vi "G# - InterfaceDemo3.vi"() -> ()   [LabVIEW 2017]
doc: "G# Interface Implementation\nThis examples demonstrates how to use the G#Interface. The interface concept is an alternative design principle to multiple inheritance (just as in C# and Java). Classes that are not related can implement the same interface and the reference of the interface could be treated just as they are from the same class.\n\nBy using the G# Debugger found in Tools->G# Debugger a text log can be followed showing how the objects were created and destroyed."
uses:
  IMyInterface2_interface/IMyInterface2.lvclass
  C:/Program Files (x86)/National Instruments/LabVIEW 2017/vi.lib/addons/_AddQ/G#Object/G#Object.lvclass
  MyClass3_class/MyClass3.lvclass
  <vilib>/addons/_AddQ/G#Object/G#Object.lvclass
  MyClass4_class/MyClass4.lvclass
panel:
  out "# of objects killed":i32
  out "OK":bool
  in  "error in (no error)":errorcluster
  out "MyClass4 is instance of IMyInterface":bool
  out "MyClass3 is instance of IMyInterface":bool
  out "error out":errorcluster
  out "Class Name":string[](array[string])
  # "G# Interface Implementation without wrapper classes using dependecy injection\nThis examples demonstrates how to use the G#Interface without using wrapper classes. It also uses dependency injection to inject the implementing class to the interface.\nThe interface concept is an alternative design principle to multiple inheritance (just as in C# and Java).\nClasses that are not related can implement the same interface and the reference of the interface could be treated just as they are from the same class.\n\nBy using the G# Debugger found in Tools->G# Debugger a text log can be followed showing how the objects were created and destroyed."
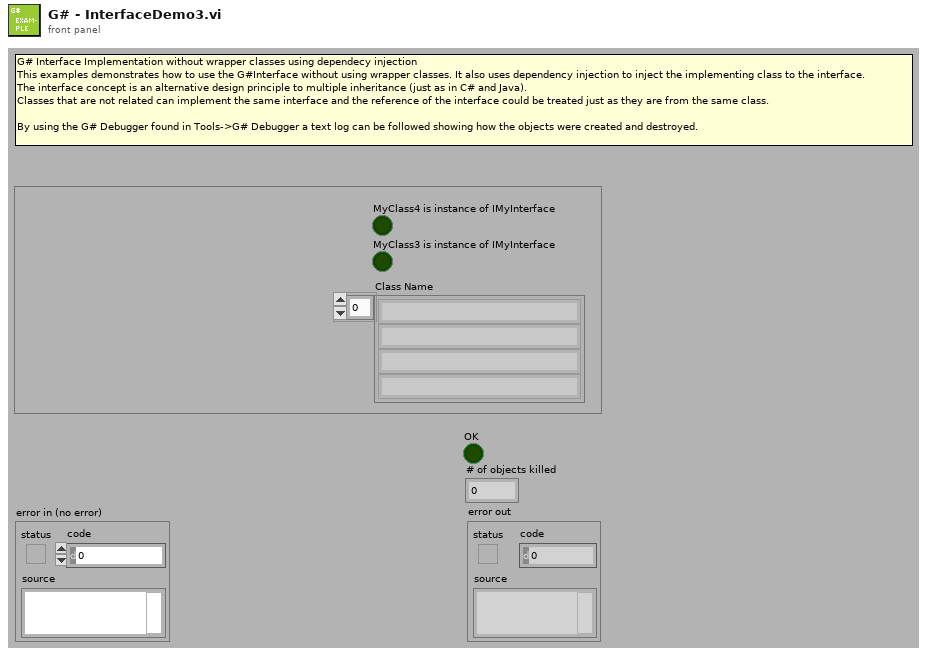
[diagram p1: front panel]
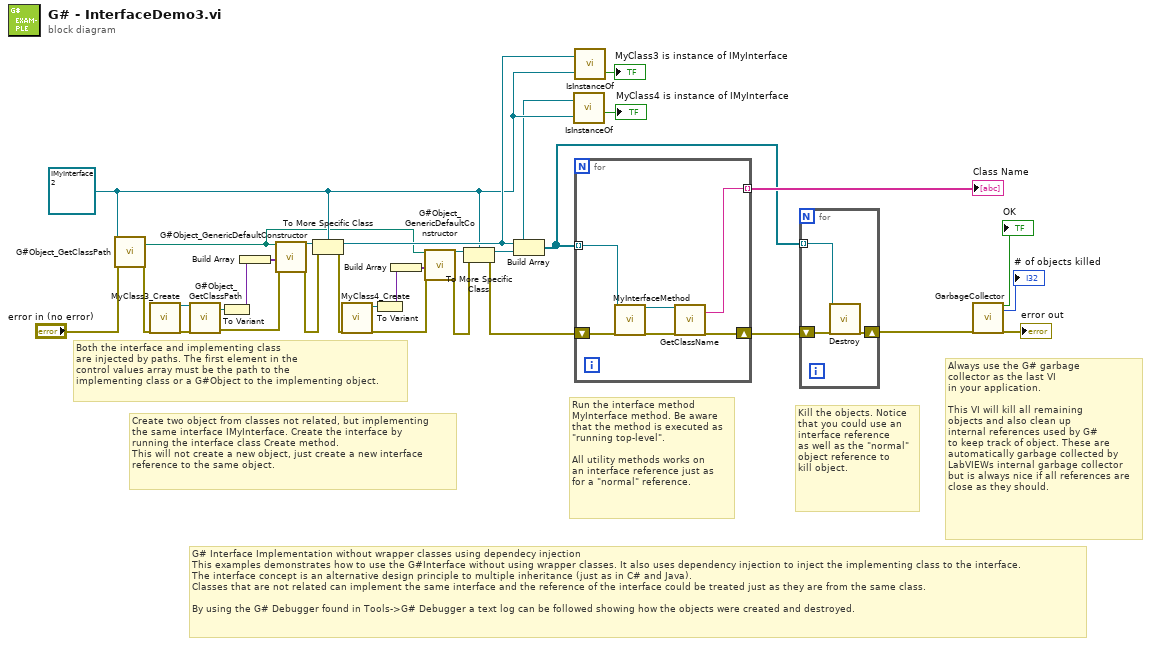
[diagram p0: block diagram]
diagram:
  w3 = refnum<class "IMyInterface2.lvclass"> refnum ("IMyInterface2.lvclass")
  # "Both the interface and implementing class\nare injected by paths. The first element in the\ncontrol values array must be the path to the\nimplementing class or a G#Object to the implementing object."
  # "G# Interface Implementation without wrapper classes using dependecy injection\nThis examples demonstrates how to use the G#Interface without using wrapper classes. It also uses dependency injection to inject the implementing class to the interface.\nThe interface concept is an alternative design principle to multiple inheritance (just as in C# and Java).\nClasses that are not related can implement the same interface and the reference of the interface could be treated just as they are from the same class.\n\nBy using the G# Debugger found in Tools->G# Debugger a text log can be followed showing how the objects were created and destroyed."
  # "Always use the G# garbage\ncollector as the last VI\nin your application.\n\nThis VI will kill all remaining\nobjects and also clean up\ninternal references used by G#\nto keep track of object. These are\nautomatically garbage collected by\nLabVIEWs internal garbage collector\nbut is always nice if all references are\nclose as they should."
  # "Kill the objects. Notice\nthat you could use an\ninterface reference\nas well as the \"normal\"\nobject reference to\nkill object."
  # "Run the interface method\nMyInterface method. Be aware\nthat the method is executed as\n\"running top-level\".\n\nAll utility methods works on\nan interface reference just as\nfor a \"normal\" reference."
  # "Create two object from classes not related, but implementing\nthe same interface IMyInterface. Create the interface by\nrunning the interface class Create method.\nThis will not create a new object, just create a new interface\nreference to the same object."
  n1 = call-dynamic "G#Object_GetClassPath.vi"("reference in"=w3, "error in (no error)"="error in (no error)") -> ("class path"=w1:path, "error out"=w21:errorcluster)  [unwired: 15 in, 1 out]
  n2 = call "MyClass3_Create.vi"("error in (no error)"=w21) -> ("reference out"=w19:refnum<class "MyClass3.lvclass">, "error out"=w20:errorcluster)  [unwired: 17 in]
  n3 = call-dynamic "G#Object_GetClassPath.vi"("reference in"=w19, "error in (no error)"=w20) -> ("class path"=w14:path, "error out"=w18:errorcluster)  [unwired: 15 in, 1 out]
  n4 = To Variant(anything=w14) -> (Variant=w12:variant)
  n5 = Build Array(w12) -> (w13:variant[])
  n6 = call <vilib>:"G#Object_GenericDefaultConstructor.vi"("class path"=w1, "control values"=w13, "error in (no error)"=w18) -> ("reference out"=w17:refnum<class "G#Object.lvclass">, "error out"=w16:errorcluster)  [unwired: 14 in, 1 out]
  n7 = To More Specific Class(target class=w3, reference=w17, error in=w16) -> (specific class reference=w10:refnum<class "IMyInterface2.lvclass">, error out=w15:errorcluster)
  n8 = call "MyClass4_Create.vi"("error in (no error)"=w15) -> ("reference out"=w8:refnum<class "MyClass4.lvclass">, "error out"=w9:errorcluster)  [unwired: 17 in]
  n9 = To Variant(anything=w8) -> (Variant=w7:variant)
  n10 = Build Array(w7) -> (w6:variant[])
  n11 = call <vilib>:"G#Object_GenericDefaultConstructor.vi"("class path"=w1, "control values"=w6, "error in (no error)"=w9) -> ("reference out"=w11:refnum<class "G#Object.lvclass">, "error out"=w5:errorcluster)  [unwired: 14 in, 1 out]
  n12 = To More Specific Class(target class=w3, reference=w11, error in=w5) -> (specific class reference=w2:refnum<class "IMyInterface2.lvclass">, error out=w4:errorcluster)
  n13 = Build Array(w10, w2) -> (w28:refnum<class "IMyInterface2.lvclass">[])
  n14 = call-dynamic "IsInstanceOf.vi"("is object instance of"=w3, "reference in"=w2) -> ("is instance of"=→"MyClass4 is instance of IMyInterface":bool)  [unwired: 1 out]
  n15 = call-dynamic "IsInstanceOf.vi"("is object instance of"=w3, "reference in"=w10) -> ("is instance of"=→"MyClass3 is instance of IMyInterface":bool)  [unwired: 1 out]
  n16 = for {
    shift-right: [w34] -> w31
    shift-left: w4 -> [w37]
    tunnel: w28 -> [w36] mode=indexing
    tunnel: [w32] -> w30 mode=indexing
    n17 = call-dynamic "MyInterfaceMethod.vi"("reference in"=w36, "error in (no error)"=w37) -> ("reference out"=w33:refnum<class "IMyInterface2.lvclass">, "error out"=w35:errorcluster)  [unwired: 16 in]
    n18 = call-dynamic "GetClassName.vi"("reference in"=w33, "error in (no error)"=w35) -> ("class name"=w32:string, "error out"=w34:errorcluster)  [unwired: 13 in, 3 out]
  }
  "Class Name" <- w30
  n19 = for {
    shift-right: [w39] -> w29
    shift-left: w31 -> [w40]
    tunnel: w28 -> [w38] mode=indexing
    n20 = call-dynamic "Destroy.vi"("reference in"=w38, "error in (no error)"=w40) -> ("error out"=w39:errorcluster)  [unwired: 16 in, 1 out]
  }
  n21 = call <vilib>:"GarbageCollector.vi"("error in (no error)"=w29) -> ("OK"=→"OK":bool, "# of objects killed"=→"# of objects killed":i32, "error out"=→"error out":errorcluster)  [unwired: 16 in]
